vi "events.vi"(9 "Debug":bool, 10 "View":string, 11 "httpRequestID":u32) -> ()   [LabVIEW 2013]
uses:
  FRCts20_EspEngine.lvlib
  <vilib>/wsapi/NI_WebServices.lvlib
  <vilib>/wsapi/subVIs/Set Boolean ESP Variable.vi
  TypeDefs/FRCts20_EspEngine_Event.ctl
  TypeDefs/FRCts20_EspEngine_Team.ctl
  TypeDefs/FRCts20_EspEngine_Universe.ctl
  Web Methods/source/VI Source/Web Method Public Interface/FRCts20_WebMethods_ctl_teamIdentifier.ctl
  Web Methods/source/VI Source/FRCts20_WebMethods.lvlib
  Backend/source/VI Source/FRCts20_Backend_API/FRCts20_Backend_API_SW.ctl
  Backend/source/VI Source/FRCts20_Backend_API/FRCts20_Backend_API.lvlib
  Web Methods/source/VI Source/Web Method Public Interface/FRCts20_WebMethods_ctl_singleTeam.ctl
  Backend/source/VI Source/FRCts20_Backend_API/FRCts20_Backend_API_Status.ctl
  Web Methods/source/VI Source/Web Method Public Interface/FRCts20_WebMethods_ctl_request.ctl
  Web Methods/source/VI Source/Web Method Public Interface/FRCts20_WebMethods_ctl_singleEvent.ctl
  Web Methods/source/VI Source/Web Method Public Interface/FRCts20_WebMethods_ctl_teams.ctl
  Web Methods/source/VI Source/Web Method Public Interface/FRCts20_WebMethods_ctl_events.ctl
panel:
  in  "Events":T1={"Live Events"=[{"Team"=[], "Issue Count"=6, "Location"="LA", "Start Date "=timestamp(0 s since 1904-01-01)}, {"Team"=[], "Issue Count"=2, "Location"="SF", "Start Date "=timestamp(0 s since 1904-01-01)}, {"Team"=[], "Issue Count"=0, "Location"="NYC", "Start Date "=timestamp(0 s since 1904-01-01)}], "Non Live Events"=[{"Team"=[], "Issue Count"=0, "Location"="Dallas", "Start Date "=timestamp(0 s since 1904-01-01)}, {"Team"=[], "Issue Count"=0, "Location"="Austin", "Start Date "=timestamp(0 s since 1904-01-01)}, {"Team"=[], "Issue Count"=0, "Location"="San Antonio", "Start Date "=timestamp(0 s since 1904-01-01)}]}
  in  "Teams":T4
  out "error out":errorcluster
  in  "Universe":T7={"TeamsListLength"=1, "Teams"=[{"Team"={"Events"=[], "Robot Name"="", "Kinect"=FALSE, "Vision"=FALSE, "Can"=FALSE, "Tags"="", "Avatar URL"="", "Team"={"Team Nickname"="", "Team Number "=0, "UniqueId"=0}, "SWType"=""}, "RequestListLength"=0, "Requests"=[]}], "LiveEventListLength"=3, "LiveEvents"=[{"Single Event"={"Team"=[], "Issue Count"=3, "Location"="SF", "Start Date "=timestamp(0 s since 1904-01-01)}, "EventOpenIssueCount"=3, "Requests"=[], "ClosedRequests"=[], "NotFoundStatus"=FALSE}, {"Single Event"={"Team"=[], "Issue Count"=2, "Location"="NYC", "Start Date "=timestamp(0 s since 1904-01-01)}, "EventOpenIssueCount"=2, "Requests"=[], "ClosedRequests"=[], "NotFoundStatus"=FALSE}, {"Single Event"={"Team"=[], "Issue Count"=0, "Location"="LA", "Start Date "=timestamp(0 s since 1904-01-01)}, "EventOpenIssueCount"=0, "Requests"=[], "ClosedRequests"=[], "NotFoundStatus"=FALSE}], "NonLiveEventListLength"=2, "NonLiveEvents"=[{"Single Event"={"Team"=[], "Issue Count"=2, "Location"="Austin", "Start Date "=timestamp(0 s since 1904-01-01)}, "EventOpenIssueCount"=2, "Requests"=[], "ClosedRequests"=[], "NotFoundStatus"=FALSE}, {"Single Event"={"Team"=[], "Issue Count"=0, "Location"="Dallas", "Start Date "=timestamp(0 s since 1904-01-01)}, "EventOpenIssueCount"=0, "Requests"=[], "ClosedRequests"=[], "NotFoundStatus"=FALSE}], "OpenIssueCount"=5, "NotFoundStatus"=FALSE}
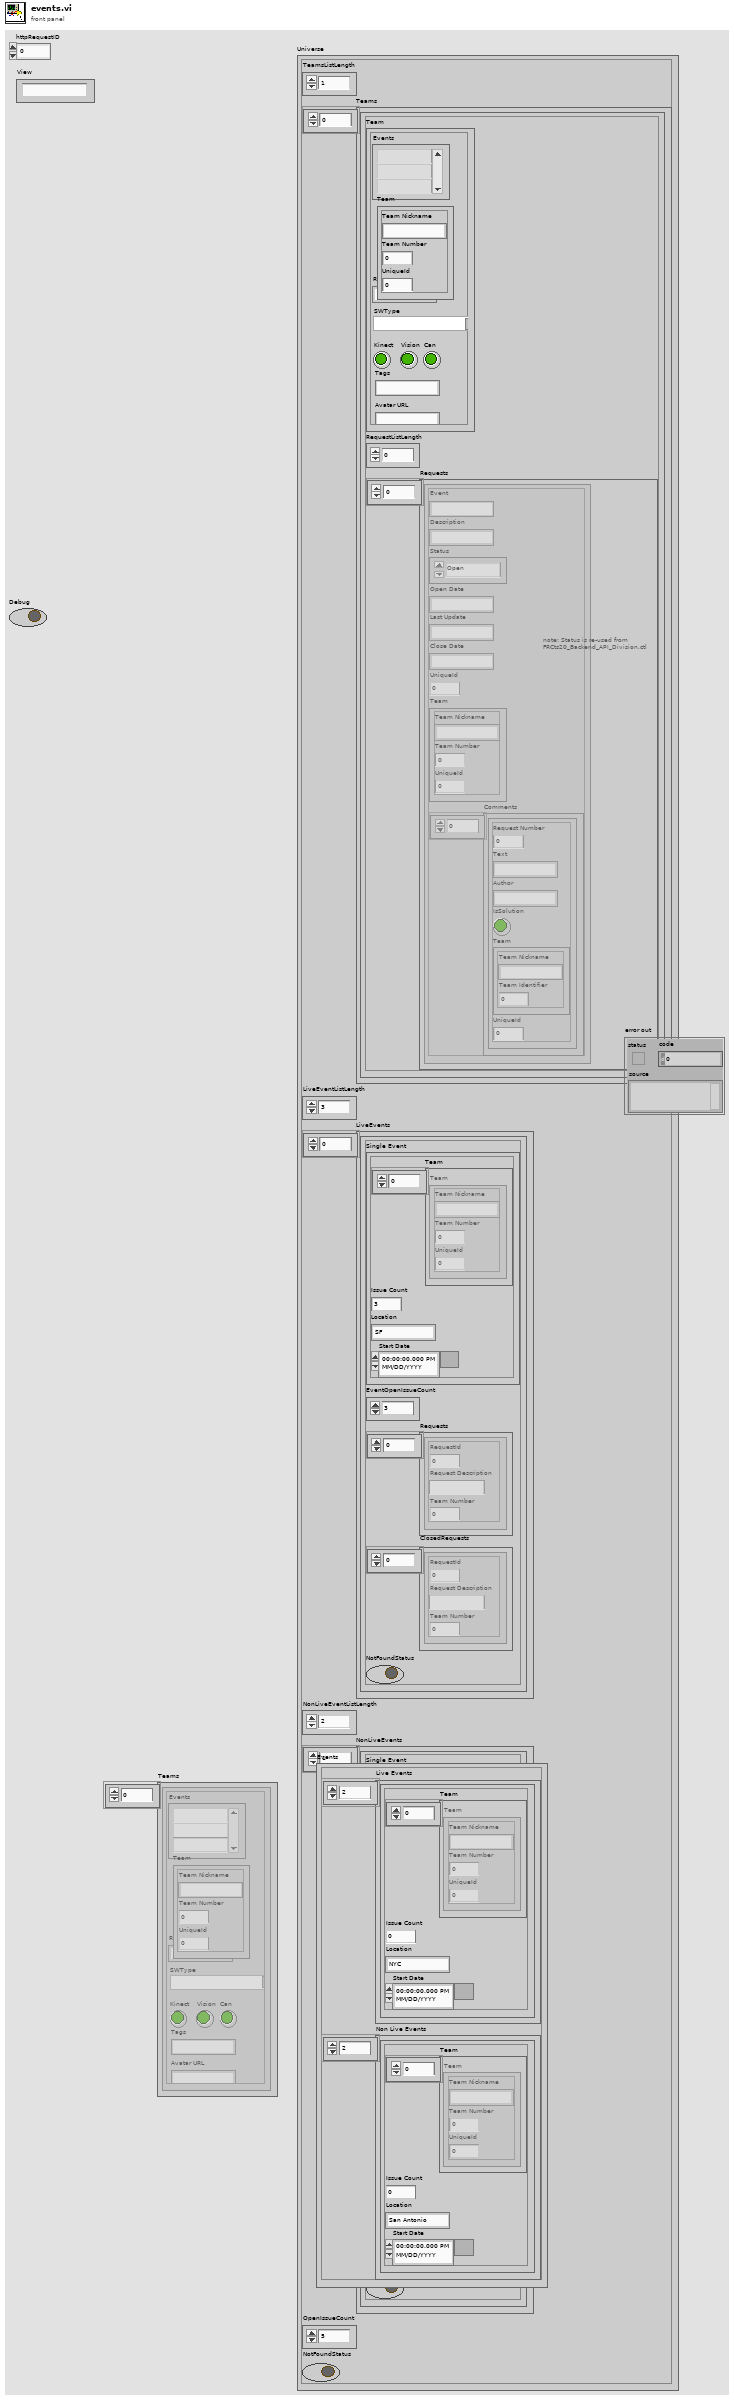
[diagram p1: front panel]
types:
  T1 = typedef "FRCts20_WebMethods.lvlib/FRCts20_WebMethods_ctl_events.ctl" = cluster{"Live Events":cluster{"Team":T2[], "Issue Count":i32, "Location":string, "Start Date ":timestamp}[], "Non Live Events":T3[]}
  T2 = typedef "FRCts20_WebMethods.lvlib/FRCts20_WebMethods_ctl_teamIdentifier.ctl" = cluster{"Team Nickname":string, "Team Number ":u32, "UniqueId":u32}
  T3 = typedef "FRCts20_WebMethods.lvlib/FRCts20_WebMethods_ctl_singleEvent.ctl" = cluster{"Team":T2[], "Issue Count":i32, "Location":string, "Start Date ":timestamp}
  T4 = typedef "FRCts20_WebMethods.lvlib/FRCts20_WebMethods_ctl_teams.ctl" = T5[]
  T5 = typedef "FRCts20_WebMethods.lvlib/FRCts20_WebMethods_ctl_singleTeam.ctl" = cluster{"Events":string[], "Robot Name":string, "Kinect":bool, "Vision":bool, "Can":bool, "Tags":string, "Avatar URL":string, "Team":T2, "SWType":T6}
  T6 = typedef "FRCts20_Backend_API.lvlib/FRCts20_Backend_API_SW.ctl" = string
  T7 = typedef "FRCts20_EspEngine.lvlib/FRCts20_EspEngine_Universe.ctl" = cluster{"TeamsListLength":i16, "Teams":T8[], "LiveEventListLength":i16, "LiveEvents":T11[], "NonLiveEventListLength":i16, "NonLiveEvents":T11[], "OpenIssueCount":i16, "NotFoundStatus":bool}
  T8 = typedef "FRCts20_EspEngine.lvlib/FRCts20_EspEngine_Team.ctl" = cluster{"Team":T5, "RequestListLength":i16, "Requests":T9[]}
  T9 = typedef "FRCts20_WebMethods.lvlib/FRCts20_WebMethods_ctl_request.ctl" = cluster{"Event":string, "Description":string, "Status":T10, "Open Date":string, "Last Update":string, "Close Date":string, "UniqueId":i32, "Team":cluster{"Team Nickname":string, "Team Number ":i32, "UniqueId":i32}, "Comments":cluster{"Request Number":dbl, "Text":string, "Author":string, "IsSolution":bool, "Team":cluster{"Team Nickname":string, "Team Identifier ":dbl}, "UniqueId":i32}[]}
  T10 = typedef "FRCts20_Backend_API.lvlib/FRCts20_Backend_API_Status.ctl" = enum16{"Open", "In Work", "Closed"}
  T11 = typedef "FRCts20_EspEngine.lvlib/FRCts20_EspEngine_Event.ctl" = cluster{"Single Event":T3, "EventOpenIssueCount":i16, "Requests":cluster{"RequestId":i32, "Request Description":string, "Team Number":i32}[], "ClosedRequests":cluster{"RequestId":i32, "Request Description":string, "Team Number":i32}[], "NotFoundStatus":bool}
  T12 = typedef "FRCts20_EspEngine.lvlib/FRCts20_EspEngine_SearchBrowser.ctl" = cluster{"Event":cluster{"Event Index":u32, "Event Name":string, "Start Time":timestamp, "End Time":timestamp, "OpenIssues":u8, "IsLive":bool}[], "select-choice-software":string, "select-choice-location":string}
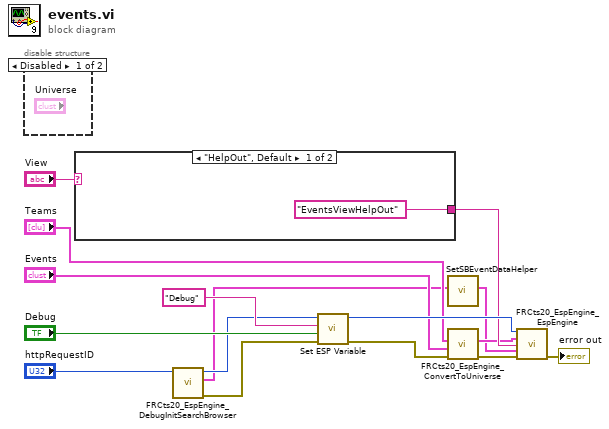
[diagram p0: block diagram]
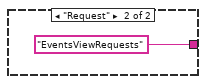
[diagram p3: hidden frame]
diagram:
  n1 = disable-structure shown="Disabled" {
    frame Disabled {
    }
    frame Enabled {
    }
  }
  n2 = case shown="\"HelpOut\", Default" "View" {
    tunnel: ["EventsViewHelpOut" "EventsViewRequests"] -> w11
    frame "HelpOut", Default {
    }
    frame "Request" {
    }
  }
  n3 = call "FRCts20_EspEngine_DebugInitSearchBrowser.vi"("httpRequestID"="httpRequestID") -> ("error out"=w3:errorcluster, "SearchBrowser"=w2:T12, "httpRequestID out"=w4:u32)  [unwired: 8 in]
  n4 = call-poly <vilib>:"Set ESP Variable.vi"("error in (no error)"=w3, "value"="Debug", "key"="Debug", "httpRequestID"=w4) -> ("error out"=w8:errorcluster, "httpRequestID out"=w14:u32)  [unwired: 6 in]
  n5 = call "SetSBEventDataHelper.vi"("SearchBrowser"=w2) -> ("SearchBrowser"=w1:T12)  [unwired: 10 in]
  n6 = call "FRCts20_EspEngine_ConvertToUniverse.vi"("error in (no error)"=w8, "Events"="Events", "Teams"="Teams") -> ("error out"=w7:errorcluster, "Universe"=w6:T7)  [unwired: 7 in]
  n7 = call "FRCts20_EspEngine_EspEngine.vi"("httpRequestID"=w14, "Cluster"=w6, "Page"=w11, "SearchBrowser"=w1, "error in (no error)"=w7) -> ("error out"=→"error out":errorcluster)  [unwired: 9 in, 1 out]
